vi "Convert to DAAG Frame Sync Clock config.vi"(11 "digital serial input settings":T1={"number of channels"=0, "data justification"=enum."Left Justified", "endianness"=enum."LSB First", "channel length"=0, "bit depth"=0, "frame clock rate"=0.0, "bit clock edge sync"=enum."Falling", "master clock source"=enum."Internal", "master clock rate"=0.0, "Logic Level"=enum."1.2 V", "frame sync edge for channel 0"=enum."Rising", "Channel 0 Offset"=0}) -> (2 "Bit Clock rate":u32=3025000 format="%.4p", 3 "Frame Sync Clock Control":T7={"Frame Length"=64, "Frame Sync Pulse Width"=32, "Bit Clock Edge  Sync"=enum."Falling"})   [LabVIEW 2022 SP3, in "digital serial input cfg file.lvlib"]
uses:
  digital serial input cfg file.lvlib
  <vilib>/PDM Acquisition Toolkit/shared/controls/PCM Frame Sync Control.ctl
  <vilib>/PDM Acquisition Toolkit/shared/controls/Digital Edge.ctl
  controls/digital serial audio/digital serial input settings.ctl
  <vilib>/PDM Acquisition Toolkit/shared/controls/PCM Data Justification.ctl
  <vilib>/PDM Acquisition Toolkit/shared/controls/PCM Bit Endianness.ctl
  controls/master clock source.ctl
  <vilib>/PDM Acquisition Toolkit/host/Classes/Session/Controls/Logic Levels.ctl
  <vilib>/PDM Acquisition Toolkit/shared/PDM Shared.lvlib
  <vilib>/PDM Acquisition Toolkit/host/Classes/Session/DecoderSession.lvclass
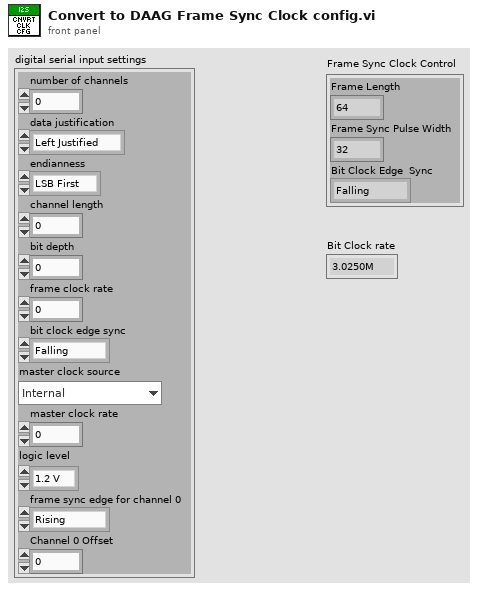
[diagram p1: front panel]
types:
  T1 = typedef "digital serial input settings.ctl" = cluster{"number of channels":u32, "data justification":T2, "endianness":T3, "channel length":u32, "bit depth":u32, "frame clock rate":dbl, "bit clock edge sync":T4, "master clock source":T5, "master clock rate":dbl, "Logic Level":T6, "frame sync edge for channel 0":T4, "Channel 0 Offset":u32}
  T2 = typedef "PDM Shared.lvlib/PCM Data Justification.ctl" = enum16{"Left Justified", "Right Justified"}
  T3 = typedef "PDM Shared.lvlib/PCM Bit Endianness.ctl" = enum16{"MSB First", "LSB First"}
  T4 = typedef "PDM Shared.lvlib/Digital Edge.ctl" = enum8{"Rising", "Falling"}
  T5 = typedef "master clock source.ctl" = enum32{"Internal", "External"}
  T6 = typedef "PDM Acquisition Class Library.lvlib/DecoderSession.lvclass/Logic Levels.ctl" = enum16{"3.3 V", "1.8 V", "1.2 V"}
  T7 = typedef "PDM Shared.lvlib/PCM Frame Sync Control.ctl" = cluster{"Frame Length":u16, "Frame Sync Pulse Width":u16, "Bit Clock Edge  Sync":T4}
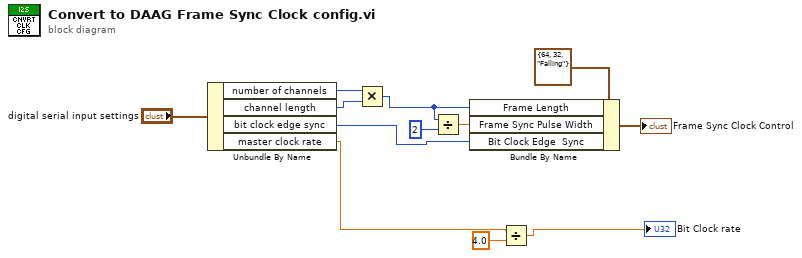
[diagram p0: block diagram]
diagram:
  n1 = Unbundle By Name("digital serial input settings") -> ("number of channels"=w6:u32, "channel length"=w5:u32, "bit clock edge sync"=w8:T4, "master clock rate"=w3:dbl)
  n2 = Multiply(x=w6, y=w5) -> (x*y=w4:u32)
  n3 = Divide(x=w4, y=u32 2) -> (x/y=w10:dbl)
  n4 = Bundle By Name(cluster=T7 {"Frame Length"=64, "Frame Sync Pulse Width"=32, "Bit Clock Edge  Sync"=enum."Falling"} ("Frame Sync Clock Control"), "Frame Length"=w4, "Frame Sync Pulse Width"=w10, "Bit Clock Edge  Sync"=w8) -> (→"Frame Sync Clock Control":T7)
  n5 = Divide(x=w3, y=4.0) -> (x/y=→"Bit Clock rate":dbl)
